vi "test_python.vi"() -> ()   [LabVIEW 2019]
panel:
  out "standard error":string
  out "error out":errorcluster
  in  "working directory":path=path ""
  out "standard output":string
  in  "command line":string="python opencv.py"
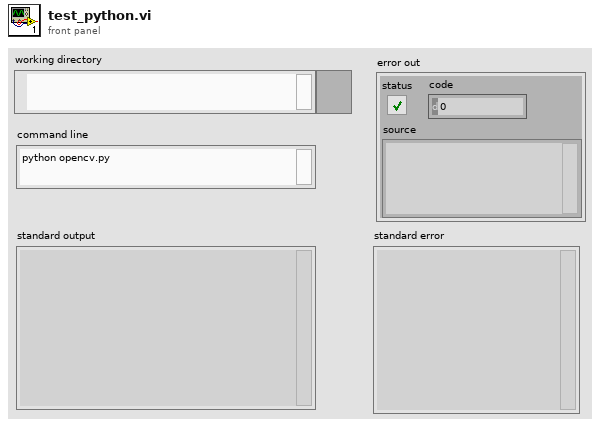
[diagram p1: front panel]
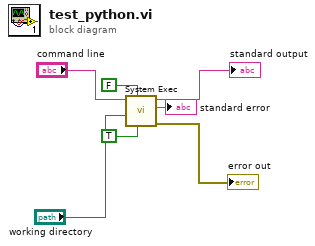
[diagram p0: block diagram]
diagram:
  n1 = call <vilib>:"System Exec.vi"("run minimized? (F)"=TRUE, "wait until completion? (T)"=FALSE, "working directory"="working directory", "command line"="command line") -> ("error out"=→"error out":errorcluster, "standard error"=→"standard error":string, "standard output"=→"standard output":string)  [unwired: 4 in, 1 out]
